vi "Autosetup.vi"(8 "error in (no error)":errorcluster, 11 "KS EDU-X 1002G in":refnum<class "KS EDU-X 1002G.lvclass">) -> (0 "error out":errorcluster, 3 "KS EDU-X 1002G out":refnum<class "KS EDU-X 1002G.lvclass">)   [LabVIEW 2020, in "Oscilloscope.lvlib" / "KS EDU-X 1002G.lvclass"]
uses:
  KS EDU-X 1002G.lvclass
  C:/Users/ronad/Osciloscopio/Osciloscopio DQMH/Libraries/Oscilloscope/Clases/Osciloscopio/Osciloscopio.lvclass
  Clases/Osciloscopio/Osciloscopio.lvclass/Osciloscopio.ctl
  Clases/Osciloscopio/Read COM.vi
  Clases/Osciloscopio/Write COM.vi
  <instrlib>/Agilent 2000 3000 X-Series/Agilent 2000 3000 X-Series.lvlib
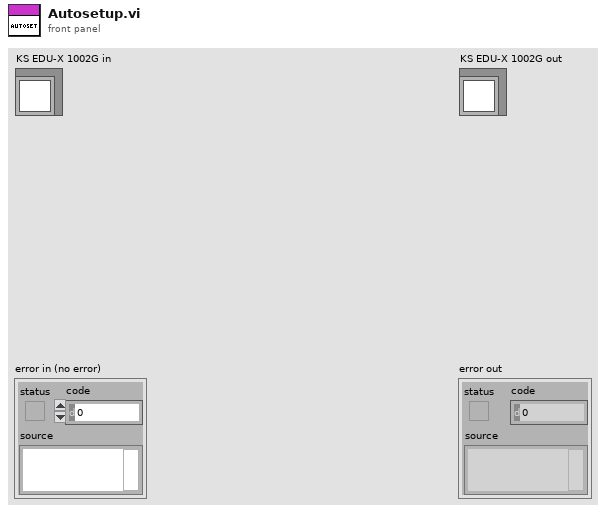
[diagram p1: front panel]
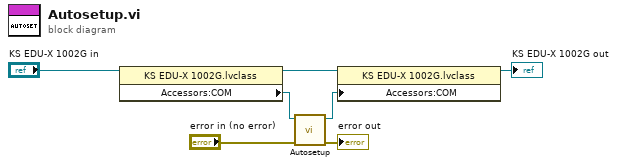
[diagram p0: block diagram]
diagram:
  n1 = property class="KS EDU-X 1002G.lvclass"(reference="KS EDU-X 1002G in") -> (reference out=w4:refnum<class "KS EDU-X 1002G.lvclass">, "Accessors:COM"=w6:refnum<visa-resource-name>)  [unwired: 1 in, 1 out]
  n2 = call <instrlib>:"Autosetup.vi"("error in (no error)"="error in (no error)", "VISA resource name"=w6) -> ("error out"=→"error out":errorcluster, "VISA resource name out"=w5:refnum<visa-resource-name>)  [unwired: 8 in]
  n3 = property class="KS EDU-X 1002G.lvclass"(reference=w4, "Accessors:COM"=w5) -> (reference out=→"KS EDU-X 1002G out":refnum<class "KS EDU-X 1002G.lvclass">)  [unwired: 1 in, 1 out]
